vi "Read_occurrence.vi"(0 "Without data DVR reference in":refnum<data-value>, 11 "error in (no error)":errorcluster) -> (4 "Without data DVR reference out":refnum<data-value>, 6 "Occurrence Ref":refnum<k4>, 15 "error out":errorcluster)   [LabVIEW 2020, in "Without Data.lvclass"]
doc: "This VI is used to read the occurrence reference from the DVR"
uses:
  Classes/Children/Intra-Application/Children/Without data/Without Data.lvclass
  Classes/Children/Intra-Application/Children/Without data/Without Data.lvclass/Without Data.ctl
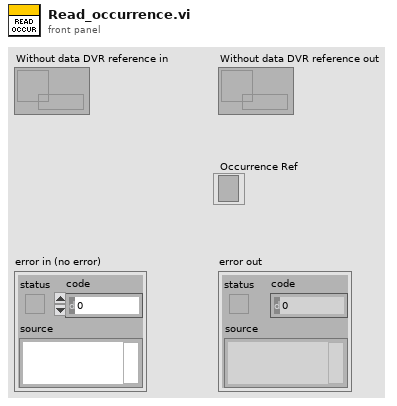
[diagram p1: front panel]
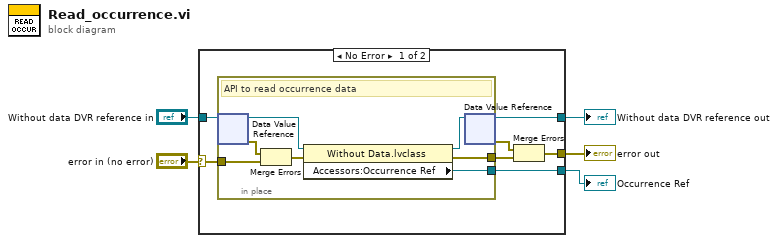
[diagram p0: block diagram]
diagram:
  n1 = case shown="No Error" "error in (no error)" {
    selector: "error in (no error)" -> [w11 w21]
    tunnel: [w7 w21] -> w4
    tunnel: "Without data DVR reference in" -> [w12 w20]
    tunnel: [w8 w20] -> w2
    tunnel: [w6 _] -> w1
    frame No Error {
      n2 = in-place "In Place Element Structure" {
        in-place-border: w11 -> [w19]
        in-place-border: [w14] -> w10
        in-place-border: [w13] -> w6
        # "API to read occurrence data"
        n3 = in-place-dvr #1(w12) -> (w16:refnum<class "Without Data.lvclass">, w18:errorcluster)
        n4 = Merge Errors(w18, w19) -> (w17:errorcluster)
        n5 = property on="Property Node" class="Without Data.lvclass"(reference=w16, error in=w17) -> (reference out=w15:refnum<class "Without Data.lvclass">, error out=w14:errorcluster, "Accessors:Occurrence Ref"=w13:refnum<k4>)
        n6 = in-place-dvr #1(w15) -> (w8:refnum<data-value>, w9:errorcluster)
      }
      n7 = Merge Errors(w9, w10) -> (w7:errorcluster)
    }
    frame Error {
    }
  }
  "error out" <- w4
  "Without data DVR reference out" <- w2
  "Occurrence Ref" <- w1
